vi "Lex Set Delimiter-Variable.vi"(8 "Error In":errorcluster) -> (0 "Error Out":errorcluster)   [LabVIEW 2018, in "Tests.lvlib" / "Lexer.lvlib"]
uses:
  Lexer.lvlib
  src/Toolkit/Low-Level/Tokens/EscapedVariable/EscapedVariable.lvclass
  src/Toolkit/Low-Level/Tokens/SetDelimiter/SetDelimiter.lvclass
  src/Toolkit/Low-Level/Support/Lex String.vi
  <vilib>/Utility/LVClass/Get LV Class Name.vi
  src/Toolkit/Low-Level/Tokens/Keyable/Keyable.lvclass
  <vilib>/addons/_JKI Toolkits/Caraya/classes/Test/Test.lvclass
  <vilib>/addons/_JKI Toolkits/Caraya/classes/Assert/Assert.lvclass
  Tests.lvlib
  src/Toolkit/Toolkit.lvlib
  src/Toolkit/Low-Level/Tokens/Abstract/Abstract.lvclass
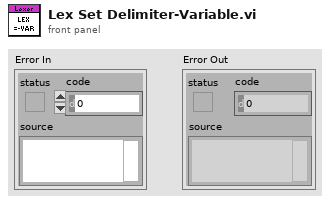
[diagram p1: front panel]
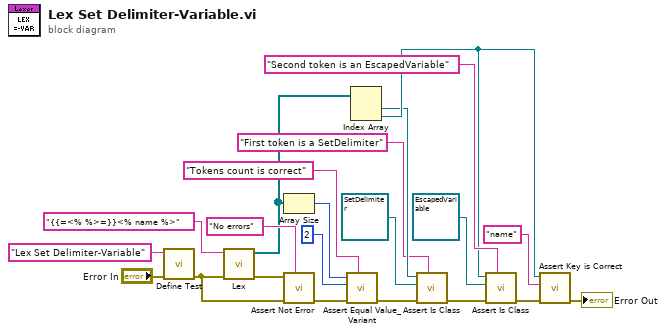
[diagram p0: block diagram]
diagram:
  n1 = call <vilib>:"Define Test.vi"("error in (no error)"="Error In", "Label (VI Title)"="Lex Set Delimiter-Variable") -> ("error out"=w8:errorcluster)  [unwired: 9 in]
  n2 = call-poly "Lex.vi"("Error In"=w8, "Input"="{{=<% %>=}}<% name %>" ("format string")) -> ("Error Out"=w20:errorcluster, "Tokens"=w14:refnum<class "Abstract.lvclass">[])  [unwired: 8 in]
  n3 = Array Size(array=w14) -> (size(s)=w16:i32)
  n4 = call <vilib>:"Assert Not Error.vi"("Label"="No errors", "error in (no error)"=w8, "Not Error?"=w20) -> ("error out"=w18:errorcluster)  [unwired: 8 in]
  n5 = call <vilib>:"Assert Equal Value_Variant.vi"("Label"="Tokens count is correct", "error in (no error)"=w18, "Y"=2 ("size(s)"), "X"=w16) -> ("error out"=w6:errorcluster)  [unwired: 7 in]
  n6 = Index Array(array=w14) -> (element #1=w2:refnum<class "Abstract.lvclass">, element #2=w3:refnum<class "Abstract.lvclass">)  [unwired: 2 in]
  n7 = call "Assert Is Class.vi"("Label"="First token is a SetDelimiter", "Error In"=w6, "Expected"=refnum<class "SetDelimiter.lvclass"> refnum ("Toolkit.lvlib:Tokens.lvlib:SetDelimiter.lvclass"), "Actual"=w2) -> ("Error Out"=w5:errorcluster)  [unwired: 7 in]
  n8 = call "Assert Is Class.vi"("Label"="Second token is an EscapedVariable", "Error In"=w5, "Expected"=refnum<class "EscapedVariable.lvclass"> refnum ("Mustache.lvlib:Tokens.lvlib:EscapedVariable.lvclass"), "Actual"=w3) -> ("Error Out"=w12:errorcluster)  [unwired: 7 in]
  n9 = call "Assert Key is Correct.vi"("Error In"=w12, "Expected"="name", "Token"=w3) -> ("Error Out"=→"Error Out":errorcluster)  [unwired: 8 in]
